vi "set_errors.vi"(0 "HGF_FGV_Visitor":refnum<class "HGF_FGV_Visitor.lvclass">, 2 "Errors":errorcluster[](array[cluster]), 3 "error":bool, 5 "error in (no error)":errorcluster) -> (14 "dup HGF_FGV_Visitor":refnum<class "HGF_FGV_Visitor.lvclass">, 19 "error out":errorcluster)   [LabVIEW 2012, in "HGF_FGV.lvlib" / "HGF_FGV_Visitor.lvclass"]
uses:
  HGF_FGV_Visitor.lvclass
  HGF_FGV_Visitor.lvclass/HGF_FGV_Visitor.ctl
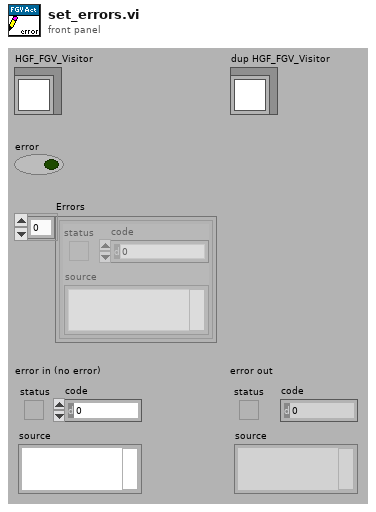
[diagram p1: front panel]
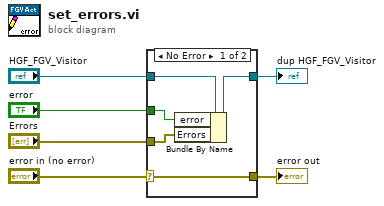
[diagram p0: block diagram]
diagram:
  n1 = case shown="No Error" "error in (no error)" {
    selector: "error in (no error)" -> [w11 w12]
    tunnel: [w11 w12] -> w5
    tunnel: [w9 w13] -> w3
    tunnel: "HGF_FGV_Visitor" -> [w10 w13]
    tunnel: "Errors" -> [w8 _]
    tunnel: "error" -> [w7 _]
    frame No Error {
      n2 = Bundle By Name(cluster=w10, "error"=w7, "Errors"=w8) -> (w9:refnum<class "HGF_FGV_Visitor.lvclass">)
    }
    frame Error {
    }
  }
  "error out" <- w5
  "dup HGF_FGV_Visitor" <- w3
